vi "PCert-ConfigPageNF-DBTellActor.vi"(6 "Timeout":i32=500, 8 "error in (no error)":errorcluster, 9 "Message Body":string, 10 "Message Header":string="Testing", 11 "ERP-ConfigPageNF in":refnum<class "PCert-ConfigPageNF.lvclass">) -> (0 "error out":errorcluster, 2 "Timed out?":bool, 3 "ERP-ConfigPageNF out":refnum<class "PCert-ConfigPageNF.lvclass">)   [LabVIEW 2013, in "PCert-ConfigPageNF.lvclass"]
uses:
  PCert-ConfigPageNF.lvclass
  PCert-ConfigPageNF.lvclass/PCert-ConfigPageNF.ctl
  ftw-dataflow/Actor/src/Connector/FTW-ActorConnector.lvclass
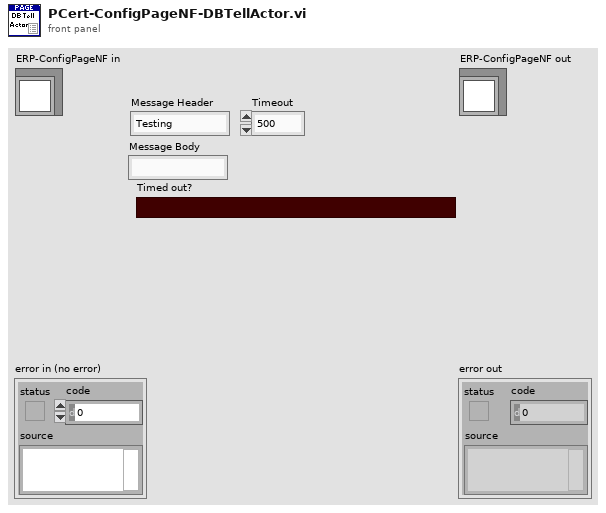
[diagram p1: front panel]
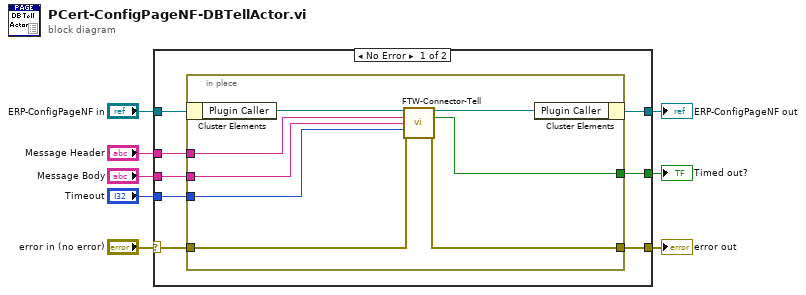
[diagram p0: block diagram]
diagram:
  n1 = case shown="No Error" "error in (no error)" {
    selector: "error in (no error)" -> [w14 w26]
    tunnel: [w9 w26] -> w7
    tunnel: [w15 w25] -> w5
    tunnel: "ERP-ConfigPageNF in" -> [w16 w25]
    tunnel: "Message Header" -> [w13 _]
    tunnel: "Message Body" -> [w12 _]
    tunnel: "Timeout" -> [w11 _]
    tunnel: [w10 _] -> w1
    frame No Error {
      n2 = in-place {
        in-place-border: w14 -> [w22]
        in-place-border: w13 -> [w21]
        in-place-border: w12 -> [w20]
        in-place-border: w11 -> [w19]
        in-place-border: [w18] -> w10
        in-place-border: [w17] -> w9
        n3 = in-place-cluster #1(w16) -> ("Plugin Caller"=w24:refnum<class "FTW-ActorConnector.lvclass">)
        n4 = call "FTW-Connector-Tell.vi"("FTW Actor Connector"=w24, "Message Header"=w21, "Message Body"=w20, "Timeout"=w19, "error in"=w22) -> ("FTW Actor Connector out"=w23:refnum<class "FTW-ActorConnector.lvclass">, "Timed out?"=w18:bool, "error out"=w17:errorcluster)  [unwired: 8 in]
        n5 = in-place-cluster #1("Plugin Caller"=w23) -> (w15:refnum<class "PCert-ConfigPageNF.lvclass">)
      }
    }
    frame Error {
    }
  }
  "error out" <- w7
  "ERP-ConfigPageNF out" <- w5
  "Timed out?" <- w1
